vi "Joystick.vi"() -> (0 "Joystick":T1)   [LabVIEW 2016]
uses:
  Global_Var-RefNum/Global_Var_Drive.vi
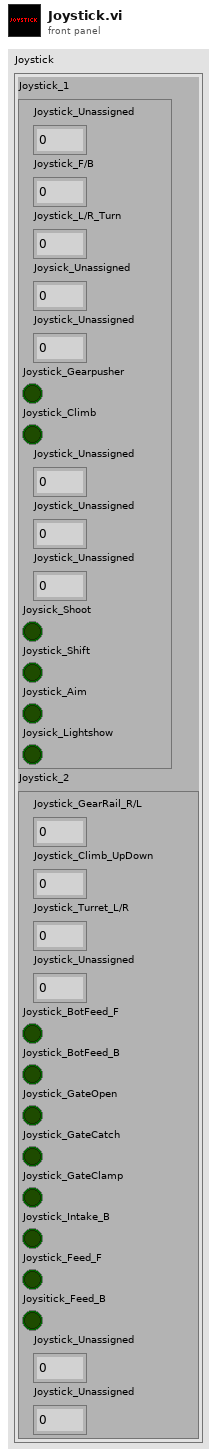
[diagram p1: front panel]
types:
  T1 = cluster{"Joystick_1":cluster{"Joystick_Unassigned":dbl, "Joystick_F/B":dbl, "Joystick_L/R_Turn":dbl, "Joysick_Unassigned":dbl, "Joystick_Unassigned":dbl, "Joystick_Gearpusher":bool, "Joystick_Climb":bool, "Joystick_Unassigned":dbl, "Joystick_Unassigned":dbl, "Joystick_Unassigned":dbl, "Joysick_Shoot":bool, "Joystick_Shift":bool, "Joystick_Aim":bool, "Joysick_Lightshow":bool}, "Joystick_2":cluster{"Joystick_GearRail_R/L":dbl, "Joystick_Climb_UpDown":dbl, "Joystick_Turret_L/R":dbl, "Joystick_Unassigned":dbl, "Joystick_BotFeed_F":bool, "Joystick_BotFeed_B":bool, "Joystick_GateOpen":bool, "Joystick_GateCatch":bool, "Joystick_GateClamp":bool, "Joystick_Intake_B":bool, "Joystick_Feed_F":bool, "Joysitick_Feed_B":bool, "Joystick_Unassigned":dbl, "Joystick_Unassigned":dbl}}
  T2 = cluster{"Joystick_Unassigned":dbl, "Joystick_F/B":dbl, "Joystick_L/R_Turn":dbl, "Joysick_Unassigned":dbl, "Joystick_Unassigned":dbl, "Joystick_Gearpusher":bool, "Joystick_Climb":bool, "Joystick_Unassigned":dbl, "Joystick_Unassigned":dbl, "Joystick_Unassigned":dbl, "Joysick_Shoot":bool, "Joystick_Shift":bool, "Joystick_Aim":bool, "Joysick_Lightshow":bool}
  T3 = cluster{"Joystick_GearRail_R/L":dbl, "Joystick_Climb_UpDown":dbl, "Joystick_Turret_L/R":dbl, "Joystick_Unassigned":dbl, "Joystick_BotFeed_F":bool, "Joystick_BotFeed_B":bool, "Joystick_GateOpen":bool, "Joystick_GateCatch":bool, "Joystick_GateClamp":bool, "Joystick_Intake_B":bool, "Joystick_Feed_F":bool, "Joysitick_Feed_B":bool, "Joystick_Unassigned":dbl, "Joystick_Unassigned":dbl}
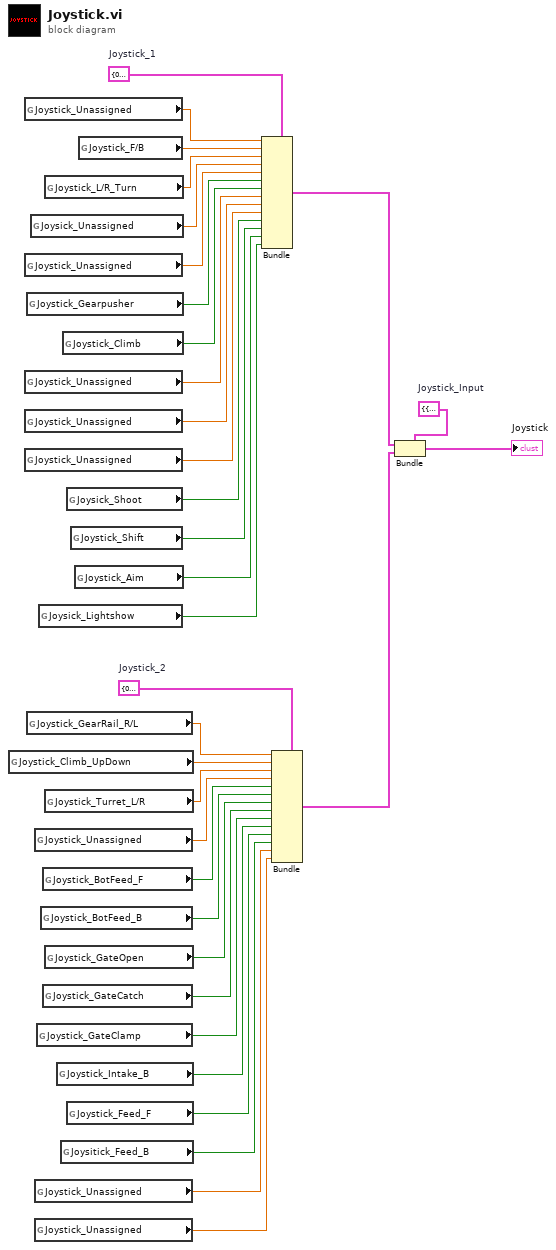
[diagram p0: block diagram]
diagram:
  w2 = T1 {"Joystick_1"={"Joystick_Unassigned"=0.0, "Joystick_F/B"=0.0, "Joystick_L/R_Turn"=0.0, "Joysick_Unassigned"=0.0, "Joystick_Unassigned"=0.0, "Joystick_Gearpusher"=FALSE, "Joystick_Climb"=FALSE, "Joystick_Unassigned"=0.0, "Joystick_Unassigned"=0.0, "Joystick_Unassigned"=0.0, "Joysick_Shoot"=FALSE, "Joystick_Shift"=FALSE, "Joystick_Aim"=FALSE, "Joysick_Lightshow"=FALSE}, "Joystick_2"={"Joystick_GearRail_R/L"=0.0, "Joystick_Climb_UpDown"=0.0, "Joystick_Turret_L/R"=0.0, "Joystick_Unassigned"=0.0, "Joystick_BotFeed_F"=FALSE, "Joystick_BotFeed_B"=FALSE, "Joystick_GateOpen"=FALSE, "Joystick_GateCatch"=FALSE, "Joystick_GateClamp"=FALSE, "Joystick_Intake_B"=FALSE, "Joystick_Feed_F"=FALSE, "Joysitick_Feed_B"=FALSE, "Joystick_Unassigned"=0.0, "Joystick_Unassigned"=0.0}}  # Joystick_Input
  w5 = T2 {"Joystick_Unassigned"=0.0, "Joystick_F/B"=0.0, "Joystick_L/R_Turn"=0.0, "Joysick_Unassigned"=0.0, "Joystick_Unassigned"=0.0, "Joystick_Gearpusher"=FALSE, "Joystick_Climb"=FALSE, "Joystick_Unassigned"=0.0, "Joystick_Unassigned"=0.0, "Joystick_Unassigned"=0.0, "Joysick_Shoot"=FALSE, "Joystick_Shift"=FALSE, "Joystick_Aim"=FALSE, "Joysick_Lightshow"=FALSE}  # Joystick_1
  w10 = T3 {"Joystick_GearRail_R/L"=0.0, "Joystick_Climb_UpDown"=0.0, "Joystick_Turret_L/R"=0.0, "Joystick_Unassigned"=0.0, "Joystick_BotFeed_F"=FALSE, "Joystick_BotFeed_B"=FALSE, "Joystick_GateOpen"=FALSE, "Joystick_GateCatch"=FALSE, "Joystick_GateClamp"=FALSE, "Joystick_Intake_B"=FALSE, "Joystick_Feed_F"=FALSE, "Joysitick_Feed_B"=FALSE, "Joystick_Unassigned"=0.0, "Joystick_Unassigned"=0.0}  # Joystick_2
  n1 = global read "Global_Var_Drive.vi" "Joystick_Climb_UpDown"() -> (w23:dbl)
  n2 = global read "Global_Var_Drive.vi" "Joystick_Unassigned"() -> (w34:dbl)
  n3 = global read "Global_Var_Drive.vi" "Joystick_Unassigned"() -> (w6:dbl)
  n4 = global read "Global_Var_Drive.vi" "Joystick_Unassigned"() -> (w9:dbl)
  n5 = global read "Global_Var_Drive.vi" "Joystick_Unassigned"() -> (w8:dbl)
  n6 = global read "Global_Var_Drive.vi" "Joystick_Unassigned"() -> (w7:dbl)
  n7 = global read "Global_Var_Drive.vi" "Joystick_Gearpusher"() -> (w30:bool)
  n8 = global read "Global_Var_Drive.vi" "Joystick_GearRail_R/L"() -> (w24:dbl)
  n9 = global read "Global_Var_Drive.vi" "Joysick_Unassigned"() -> (w31:dbl)
  n10 = global read "Global_Var_Drive.vi" "Joystick_Unassigned"() -> (w21:dbl)
  n11 = global read "Global_Var_Drive.vi" "Joystick_Unassigned"() -> (w12:dbl)
  n12 = global read "Global_Var_Drive.vi" "Joystick_Unassigned"() -> (w11:dbl)
  n13 = global read "Global_Var_Drive.vi" "Joystick_GateClamp"() -> (w16:bool)
  n14 = global read "Global_Var_Drive.vi" "Joysick_Lightshow"() -> (w25:bool)
  n15 = global read "Global_Var_Drive.vi" "Joystick_BotFeed_B"() -> (w19:bool)
  n16 = global read "Global_Var_Drive.vi" "Joystick_BotFeed_F"() -> (w20:bool)
  n17 = global read "Global_Var_Drive.vi" "Joystick_GateCatch"() -> (w17:bool)
  n18 = global read "Global_Var_Drive.vi" "Joystick_L/R_Turn"() -> (w32:dbl)
  n19 = global read "Global_Var_Drive.vi" "Joystick_Turret_L/R"() -> (w22:dbl)
  n20 = global read "Global_Var_Drive.vi" "Joystick_GateOpen"() -> (w18:bool)
  n21 = global read "Global_Var_Drive.vi" "Joystick_Intake_B"() -> (w15:bool)
  n22 = global read "Global_Var_Drive.vi" "Joysitick_Feed_B"() -> (w13:bool)
  n23 = global read "Global_Var_Drive.vi" "Joystick_Climb"() -> (w29:bool)
  n24 = global read "Global_Var_Drive.vi" "Joysick_Shoot"() -> (w28:bool)
  n25 = global read "Global_Var_Drive.vi" "Joystick_Feed_F"() -> (w14:bool)
  n26 = global read "Global_Var_Drive.vi" "Joystick_Shift"() -> (w27:bool)
  n27 = global read "Global_Var_Drive.vi" "Joystick_Aim"() -> (w26:bool)
  n28 = global read "Global_Var_Drive.vi" "Joystick_F/B"() -> (w33:dbl)
  n29 = Bundle(cluster=w5, "Joystick_Unassigned"=w34, "Joystick_F/B"=w33, "Joystick_L/R_Turn"=w32, "Joysick_Unassigned"=w31, "Joystick_Unassigned"=w6, "Joystick_Gearpusher"=w30, "Joystick_Climb"=w29, "Joystick_Unassigned"=w9, "Joystick_Unassigned"=w8, "Joystick_Unassigned"=w7, "Joysick_Shoot"=w28, "Joystick_Shift"=w27, "Joystick_Aim"=w26, "Joysick_Lightshow"=w25) -> (w3:T2)
  n30 = Bundle(cluster=w10, "Joystick_GearRail_R/L"=w24, "Joystick_Climb_UpDown"=w23, "Joystick_Turret_L/R"=w22, "Joystick_Unassigned"=w21, "Joystick_BotFeed_F"=w20, "Joystick_BotFeed_B"=w19, "Joystick_GateOpen"=w18, "Joystick_GateCatch"=w17, "Joystick_GateClamp"=w16, "Joystick_Intake_B"=w15, "Joystick_Feed_F"=w14, "Joysitick_Feed_B"=w13, "Joystick_Unassigned"=w12, "Joystick_Unassigned"=w11) -> (w4:T3)
  n31 = Bundle(cluster=w2, "Joystick_1"=w3, "Joystick_2"=w4) -> (→"Joystick":T1)
